vi "2D Helmholtz PDE Rendering (Polygon Domain).vi"(0 "PDE in":refnum<class "NI_PDE.lvclass">, 1 "plot style":T1=1 items=["Wireframe", "Polygons"], 5 "U(x, y)":dbl[](array[numeric]), 7 "Grid Points":cluster{"X":dbl, "Y":dbl}[](array[cluster]), 11 "error in (no error)":errorcluster) -> (4 "PDE out":refnum<class "NI_PDE.lvclass">, 6 "PDE Plot":refnum<vi>, 8 "Triangulation Plot":cluster{"X":dbl[], "U(x, y)":dbl[]}[](graph), 15 "error out":errorcluster)   [LabVIEW 2017, in "NI_PDE.lvlib"]
doc: "Renders the solution of the partial differential equation. You must manually select the polymorphic instance to use."
uses:
  <vilib>/gmath/NI_PDE.lvlib
  <vilib>/gmath/pde.llb/PDEClass/NI_PDE.lvclass
  <vilib>/gmath/pde.llb/Common/PDE_Plot Style.ctl
  <vilib>/gmath/pde.llb/PDEClass/PDE_Helmholtz_2D/NI_PDE_Helmholtz_2D.lvclass
  e:/builds/penguin/labview/branches/2017/dev/dist/vi.lib/gmath/pde.llb/PDEClass/NI_PDE.lvclass
  <vilib>/gmath/pde.llb/DomainClass/Domain_Steady_2D_Polygon/NI_Domain_Steady_2D_Polygon.lvclass
  e:/builds/penguin/labview/branches/2017/dev/dist/vi.lib/gmath/pde.llb/DomainClass/NI_Domain.lvclass
  <vilib>/gmath/pde.llb/DomainClass/Domain_Steady_2D_Polygon/Domain Data.ctl
  <vilib>/picture/3D Picture Control/Object/Create Object (name).vi
  <vilib>/picture/3D Picture Control/NI_3D Picture Control.lvlib
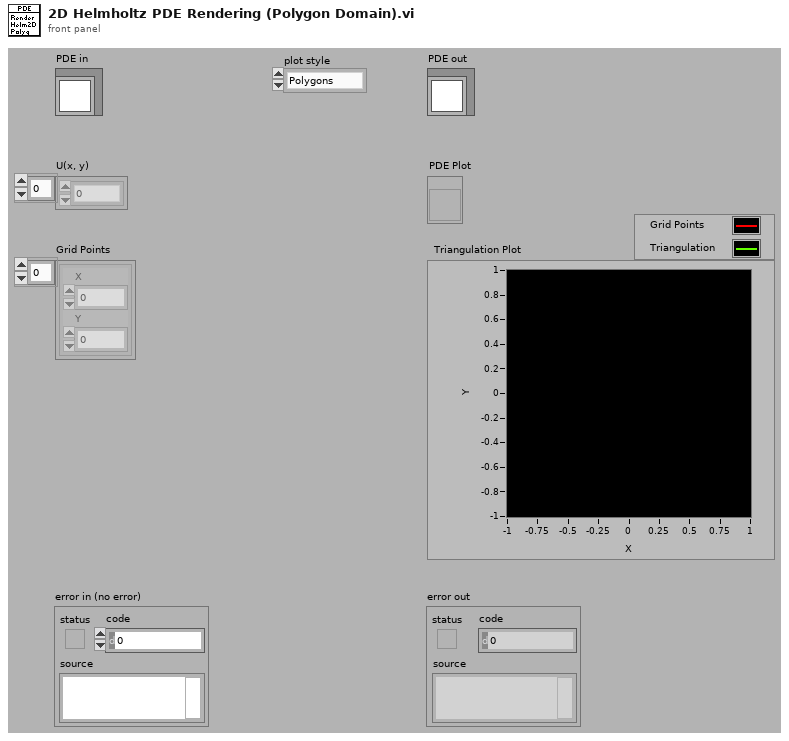
[diagram p1: front panel]
types:
  T1 = typedef "NI_PDE.lvlib/PDE_Plot Style.ctl" = i32
  T2 = typedef "NI_PDE.lvlib/NI_Domain_Steady_2D_Polygon.lvclass/Domain Data.ctl" = cluster{"X":dbl[], "Y":dbl[], "Xi":dbl[], "Yi":dbl[], "grid factor":dbl, "Triangulation":i32[][]}
  T3 = enum16{"Inherit Value", "Points", "Wireframe", "Polygons"}
  T4 = enum16{"Overall", "Per Primitive", "Per Vertex", "Binding Off"}
  T5 = enum16{"Points", "Lines", "Line Strip", "Line Loop", "Triangles", "Triangle Strip", "Triangle Fan", "Quads", "Quad Strip", "Polygon"}
  T6 = typedef "LVRGBAColorTypeDef.ctl" = cluster{"Red":sgl, "Green":sgl, "Blue":sgl, "Alpha":sgl}
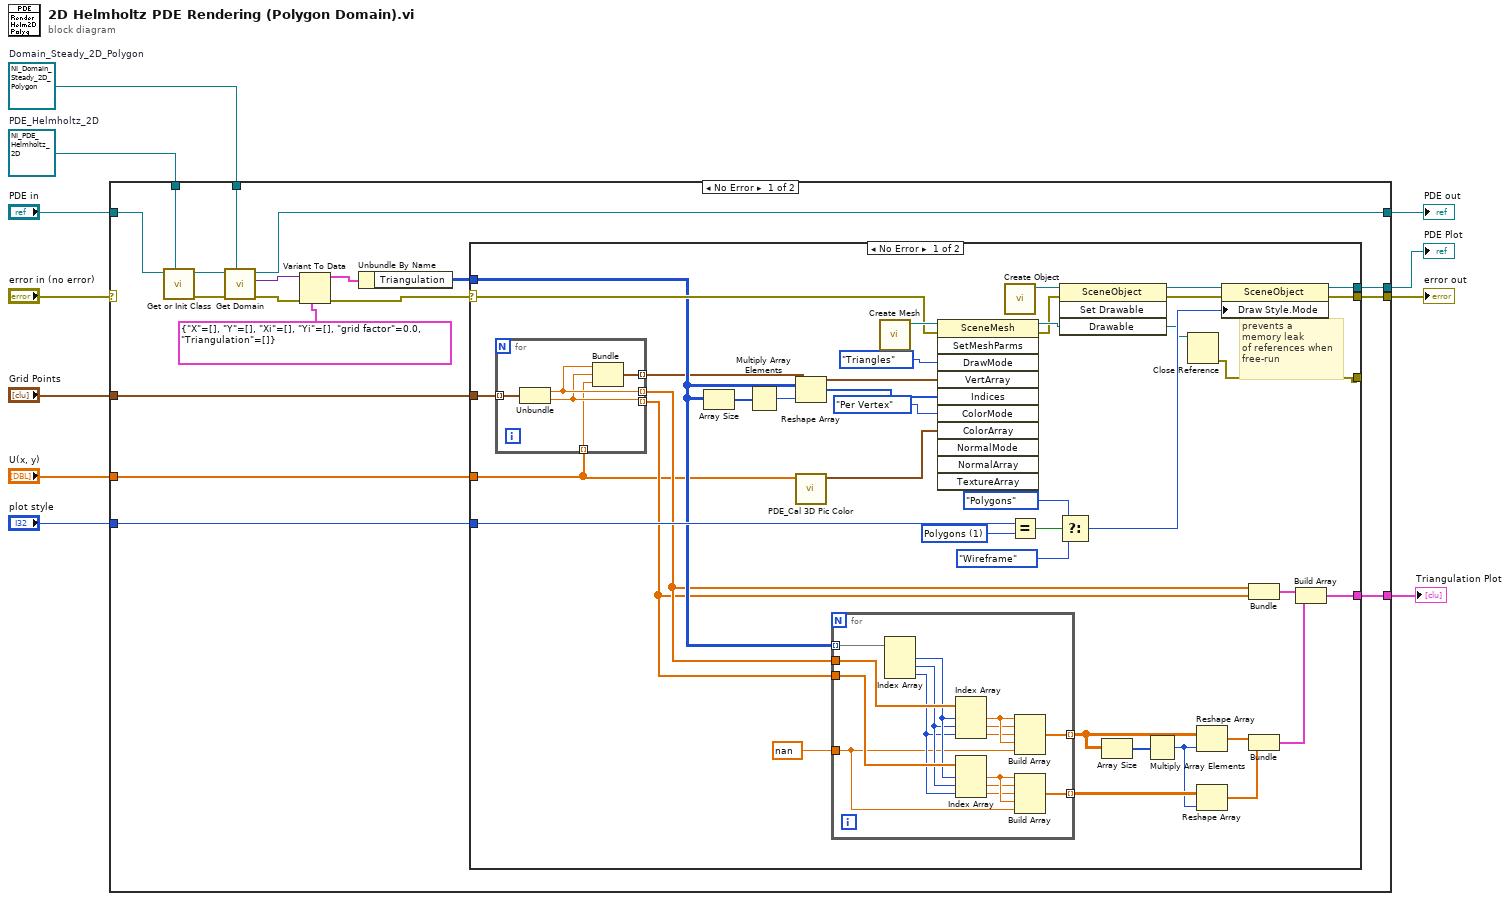
[diagram p0: block diagram]
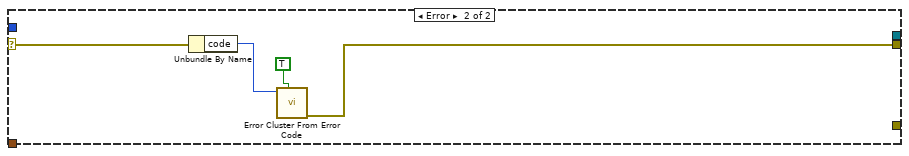
[diagram p2: hidden frame]
diagram:
  w1 = refnum<class "NI_Domain_Steady_2D_Polygon.lvclass"> refnum  # Domain_Steady_2D_Polygon
  w2 = refnum<class "NI_PDE_Helmholtz_2D.lvclass"> refnum  # PDE_Helmholtz_2D
  n1 = case shown="No Error" "error in (no error)" {
    selector: "error in (no error)" -> [_ w94]
    tunnel: "U(x, y)" -> [w29 _]
    tunnel: [w28 _] -> w10
    tunnel: [w27 w94] -> w9
    tunnel: "plot style" -> [w26 _]
    tunnel: [w25 _] -> w7
    tunnel: [w23 w93] -> w6
    tunnel: "Grid Points" -> [w24 _]
    tunnel: "PDE in" -> [w12 w93]
    tunnel: w2 -> [w14 _]
    tunnel: w1 -> [w13 _]
    frame No Error {
      n2 = call <vilib>:"Get or Init Class.vi"("target PDE"=w14, "PDE in"=w12) -> ("error out"=w16:errorcluster, "PDE out"=w15:refnum<class "NI_PDE.lvclass">)  [unwired: 1 in, 7 out]
      n3 = call <vilib>:"Get Domain.vi"("target Domain"=w13, "error in (no error)"=w16, "PDE in"=w15) -> ("error out"=w21:errorcluster, "domain"=w22:variant, "PDE out"=w23:refnum<class "NI_PDE.lvclass">)  [unwired: 6 out]
      n4 = Variant To Data(error in=w21, type=T2 {"X"=[], "Y"=[], "Xi"=[], "Yi"=[], "grid factor"=0.0, "Triangulation"=[]} ("domain data"), Variant=w22) -> (data=w18:T2, error out=w20:errorcluster)
      n5 = Unbundle By Name(w18) -> ("Triangulation"=w17:i32[][])
      n6 = case shown="No Error" w20 {
        selector: w20 -> [w55 w90]
        tunnel: w29 -> [w34 _]
        tunnel: w17 -> [w47 _]
        tunnel: [w56 _] -> w28
        tunnel: [w54 w89] -> w27
        tunnel: w26 -> [w53 _]
        tunnel: [w38 _] -> w25
        tunnel: w24 -> [w37 _]
        tunnel: [w30 _] -> _
        frame No Error {
          w32 = T1 1 items=["Wireframe", "Polygons"] ("plot style")
          # "prevents a\nmemory leak\nof references when\nfree-run"
          n7 = for {
            tunnel: w37 -> [w73] mode=indexing
            tunnel: [w72] -> w36 mode=indexing
            tunnel: [w71] -> w35 mode=indexing
            tunnel: w34 -> [w70] mode=indexing
            tunnel: [w69] -> w33 mode=indexing
            n8 = Unbundle(w73) -> ("X"=w72:dbl, "Y"=w71:dbl)
            n9 = Bundle("X"=w72, "Y"=w71, "Numeric"=w70) -> (w69:cluster{"X":dbl, "Y":dbl, "Numeric":dbl})  [unwired: 1 out]
          }
          n10 = Array Size(array=w47) -> (size(s)=w64:i32[])
          n11 = Multiply Array Elements(1:w64) -> (0:w63:i32)
          n12 = Reshape Array(w47, w63) -> (w62:i32[])
          n13 = call <vilib>:"PDE_Cal 3D Pic Color.vi"("U(x, y)"=w34) -> ("Color Array"=w57:T6[])  [unwired: 10 out]
          n14 = for {
            tunnel: w47 -> [w87] mode=indexing
            tunnel: w36 -> [w88]
            tunnel: w35 -> [w86]
            tunnel: nan -> [w80]
            tunnel: [w82] -> w45 mode=indexing
            tunnel: [w81] -> w44 mode=indexing
            n15 = Index Array(array=w87) -> (element #1=w85:i32, element #2=w84:i32, element #3=w83:i32)  [unwired: 3 in]
            n16 = Index Array(array=w88, index #1=w85, index #2=w84, index #3=w83) -> (element #1=w79:dbl, element #2=w78:dbl, element #3=w77:dbl)
            n17 = Index Array(array=w86, index #1=w85, index #2=w84, index #3=w83) -> (element #1=w76:dbl, element #2=w75:dbl, element #3=w74:dbl)
            n18 = Build Array(w79, w78, w77, w79, w80) -> (w82:dbl[])
            n19 = Build Array(w76, w75, w74, w76, w80) -> (w81:dbl[])
          }
          n20 = call <vilib>:"Create Mesh.vi"() -> ("New Mesh Refnum"=w68:refnum<vi>)  [unwired: 1 in, 10 out]
          n21 = invoke class="SceneMesh" method="SetMeshParms"(reference=w68, error in=w55, "DrawMode"=T5."Triangles" ("Draw Mode"), "VertArray"=w33, "Indices"=w62, "ColorMode"=T4."Per Vertex" ("Color Binding Mode"), "ColorArray"=w57) -> (reference out=w66:refnum<vi>, error out=w58:errorcluster)  [unwired: 4 in, 9 out]
          n22 = call-poly <vilib>:"Create Object.vi"() -> ("Scene:New Object"=w67:refnum<vi>)  [unwired: 10 in, 1 out]
          n23 = Equal?(x=w53, y=w32) -> (x = y?=w52:bool)
          n24 = invoke class="SceneObject" method="Set Drawable"(reference=w67, error in=w58, "Drawable"=w66) -> (reference out=w65:refnum<vi>, error out=w59:errorcluster, "Drawable"=w31:refnum<vi>)  [unwired: 1 in, 1 out]
          n25 = Select(t=T3."Polygons" ("Draw Style:Mode"), s=w52, f=T3."Wireframe" ("Draw Style:Mode")) -> (s? t:f=w49:T3)
          n26 = Array Size(array=w45) -> (size(s)=w46:i32[])
          n27 = Multiply Array Elements(1:w46) -> (0:w43:i32)
          n28 = Close Reference(reference=w31) -> (error out=w30:errorcluster)  [unwired: 1 in]
          n29 = Reshape Array(w45, w43) -> (w42:dbl[])
          n30 = Reshape Array(w44, w43) -> (w41:dbl[])
          n31 = property class="SceneObject"(reference=w65, error in=w59, "Draw Style.Mode"=w49) -> (reference out=w56:refnum<vi>, error out=w54:errorcluster)
          n32 = Bundle(w36, w35) -> (w40:cluster{dbl[], dbl[]})  [unwired: 1 out]
          n33 = Bundle(w42, w41) -> (w39:cluster{dbl[], dbl[]})  [unwired: 1 out]
          n34 = Build Array(w40, w39) -> (w38:cluster{dbl[], dbl[]}[])
        }
        frame Error {
          n35 = Unbundle By Name(w90) -> ("code"=w92:i32)
          n36 = call <vilib>:"Error Cluster From Error Code.vi"("show call chain? (False)"=TRUE, "error code (0)"=w92) -> ("error out"=w89:errorcluster)  [unwired: 1 in, 6 out]
        }
      }
    }
    frame Error {
    }
  }
  "PDE out" <- w6
  "error out" <- w9
  "PDE Plot" <- w10
  "Triangulation Plot" <- w7
